vi "ZenCAM Output.vi"(8 "error in (no error)":errorcluster, 9 "Output Data":T1, 10 "State":string, 11 "Camera Controller in":refnum<class "Camera Controller.lvclass">) -> (0 "error out":errorcluster, 3 "Camera Controller out":refnum<class "Camera Controller.lvclass">)   [LabVIEW 2019, in "Camera Controller.lvlib" / "Camera Controller.lvclass"]
uses:
  Camera Controller.lvclass
  <vilib>/ActorFramework/Actor/Actor.lvclass
  <vilib>/vision/Image Controls.llb/IMAQ Image.ctl
  Rack Controller/Rack Controller Messages/CameraOpticsDiagnosticsResult_RC Msg/Camera Optics Diagnostics Result_RC Msg.lvclass
  Rack Controller/Rack Controller Messages/Acknowledgement_RC Msg/Acknowledgement_RC Msg.lvclass
  Rack Controller/Rack Controller Messages/Clear_RC Msg/Clear_RC Msg.lvclass
  Algorithm/Algorithm Messages/ImagesAndCount_Algo Msg/ImagesAndCount_Algo Msg.lvclass
  Rack Controller/Rack Controller Messages/Global Count Value Change_RC Msg/Current Trigger Count_RC Msg.lvclass
  Rack Controller/Rack Controller Messages/Camera Info_RC Msg/Camera Info_RC Msg.lvclass
  Rack Controller/Rack Controller Messages/SensorDiagnosticsResult_RC Msg/SensorDiagnosticsResult_RC Msg.lvclass
  Rack Controller/Rack Controller Messages/Error Message_RC Msg/Error Message_RC Msg.lvclass
  C:/Program Files/National Instruments/LabVIEW 2019/vi.lib/ActorFramework/Actor/Actor.lvclass
  <vilib>/ActorFramework/Message Enqueuer/Message Enqueuer.lvclass
  TypeDef/Output Data.ctl
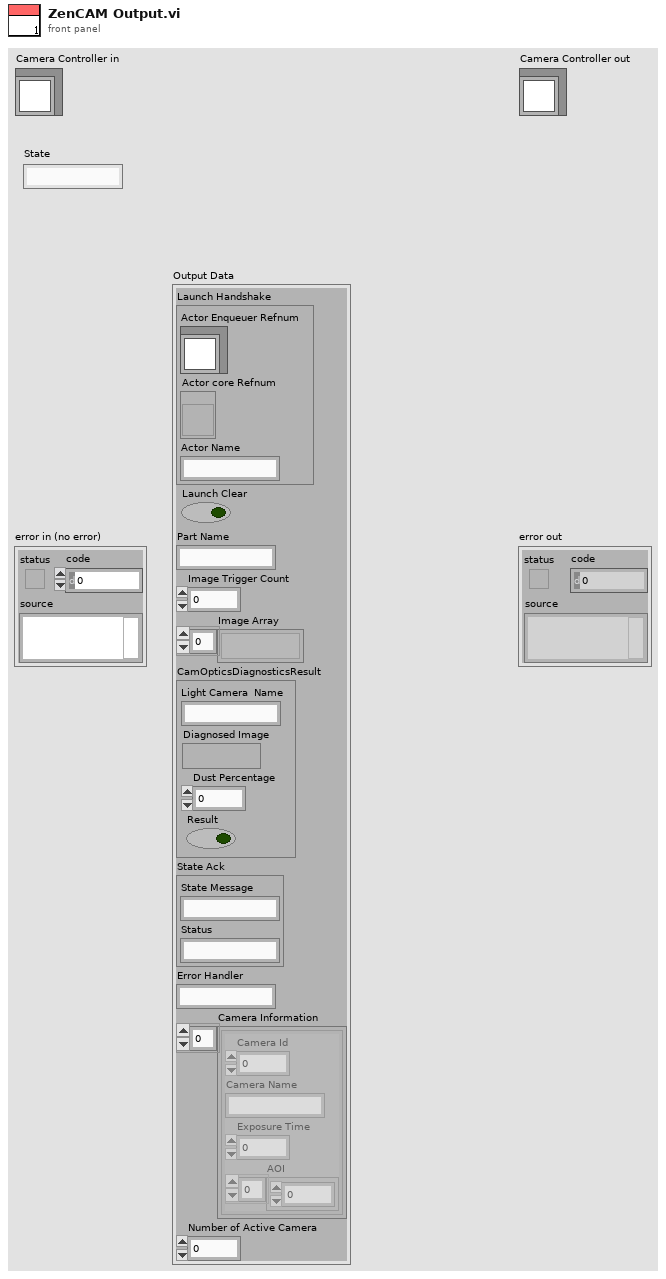
[diagram p1: front panel]
types:
  T1 = typedef "Camera Controller.lvlib/Camera Controller.lvclass/Output Data.ctl" = cluster{"Launch Handshake":cluster{"Actor Enqueuer Refnum":refnum<class "Message Enqueuer.lvclass">, "Actor core Refnum":refnum<vi>, "Actor Name":string}, "Launch Clear":bool, "Part Name":string, "Image Trigger Count":u64, "Image Array":T2[], "CamOpticsDiagnosticsResult":cluster{"Light Camera  Name":string, "Diagnosed Image":T2, "Dust Percentage":dbl, "Result":bool}, "State Ack":cluster{"State Message":string, "Status":string}, "Error Handler":string, "Camera Information":cluster{"Camera Id":i32, "Camera Name":string, "Exposure Time":i32, "AOI":i32[]}[], "Number of Active Camera":i32}
  T2 = typedef "IMAQ Image.ctl" = refnum<image>
  T3 = cluster{"Camera Names":string[], "No. of Active Cameras":u8}
  T4 = cluster{"Actor Enqueuer Refnum":refnum<class "Message Enqueuer.lvclass">, "Actor core Refnum":refnum<vi>, "Actor Name":string}
  T5 = cluster{"Camera Id":i32, "Camera Name":string, "Exposure Time":i32, "AOI":i32[]}[]
  T6 = cluster{"Light Camera  Name":string, "Diagnosed Image":T2, "Dust Percentage":dbl, "Result":bool}
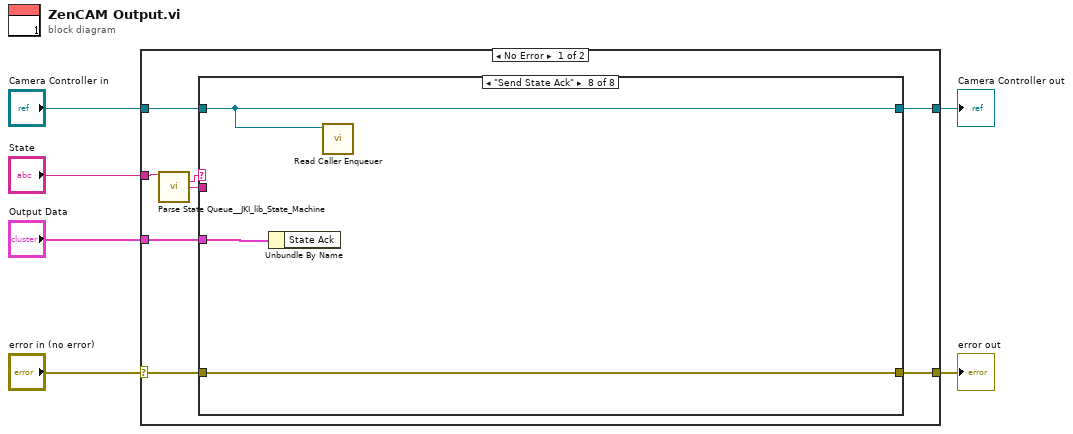
[diagram p0: block diagram]
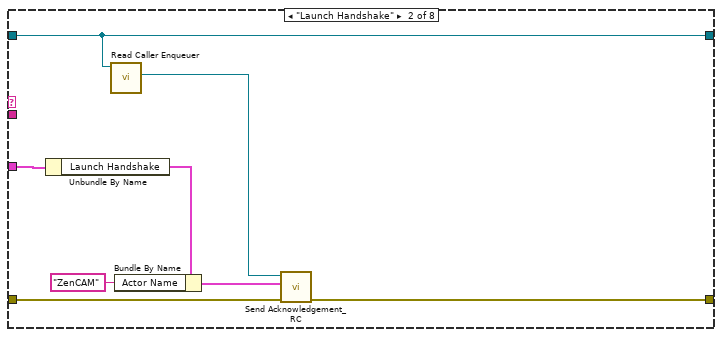
[diagram p3: hidden frame]
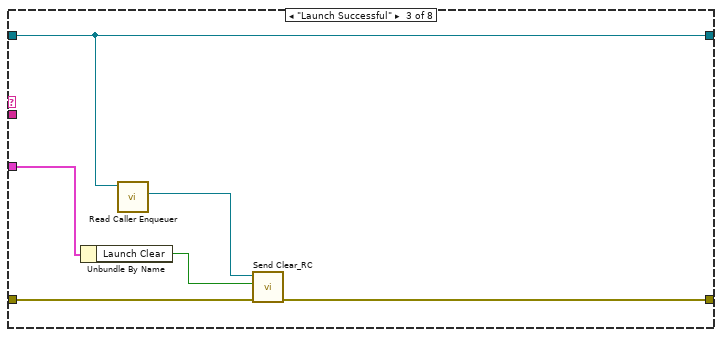
[diagram p4: hidden frame]
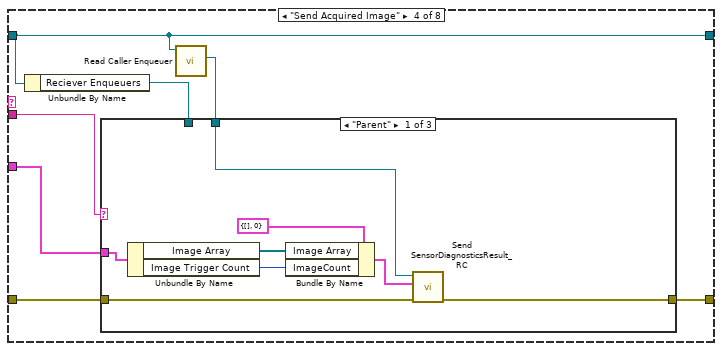
[diagram p5: hidden frame]
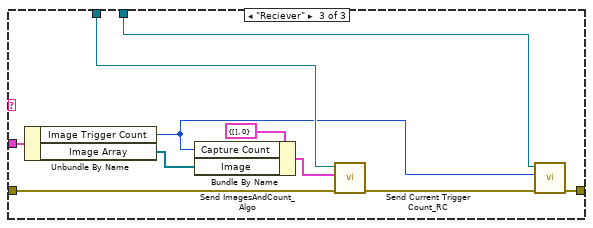
[diagram p7: hidden frame]
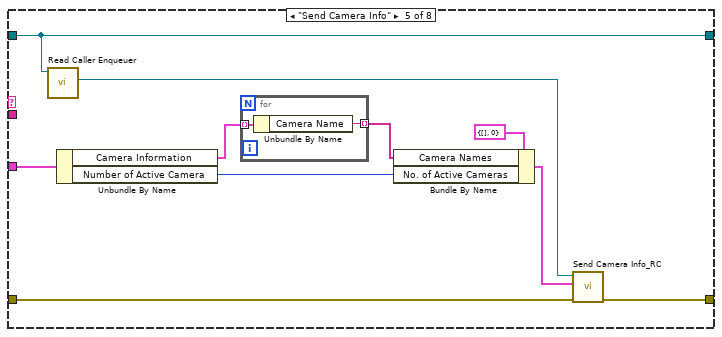
[diagram p8: hidden frame]
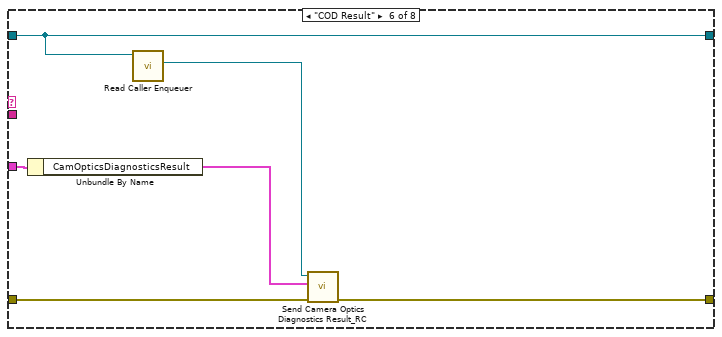
[diagram p9: hidden frame]
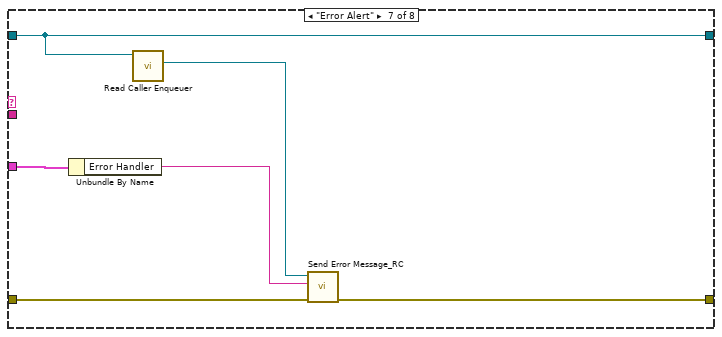
[diagram p10: hidden frame]
diagram:
  n1 = case shown="No Error" "error in (no error)" {
    selector: "error in (no error)" -> [w11 w85]
    tunnel: [w10 w85] -> w5
    tunnel: [w12 w84] -> w3
    tunnel: "Camera Controller in" -> [w13 w84]
    tunnel: "State" -> [w9 _]
    tunnel: "Output Data" -> [w14 _]
    frame No Error {
      n2 = call <vilib>:"Parse State Queue__JKI_lib_State_Machine.vi"("State Queue"=w9) -> ("Current State"=w8:string, "Arguments"=w7:string)  [unwired: 12 in, 1 out]
      n3 = case shown="\"Send State Ack\"" w8 {
        tunnel: w14 -> [_ w24 w30 w37 w66 w74 w80 w83]
        tunnel: w11 -> [w15 w21 w26 w35 w58 w72 w76 w81]
        tunnel: w13 -> [w16 w23 w29 w32 w61 w73 w79 w82]
        tunnel: [w16 w23 w29 w32 w61 w73 w79 w82] -> w12
        tunnel: [w15 w20 w25 w34 w57 w69 w75 w81] -> w10
        tunnel: w7 -> [_ _ _ w33 _ _ _ _]
        frame Default {
        }
        frame "Launch Handshake" {
          n4 = Unbundle By Name(w24) -> ("Launch Handshake"=w19:T4)
          n5 = call <vilib>:"Read Caller Enqueuer.vi"("Actor"=w23) -> ("Caller Enqueuer"=w22:refnum<class "Message Enqueuer.lvclass">)  [unwired: 10 in]
          n6 = Bundle By Name(cluster=w19, "Actor Name"="ZenCAM") -> (w18:T4)
          n7 = call "Send Acknowledgement_RC.vi"("error in (no error)"=w21, "Acknowledgement_RC"=w18, "Message Enqueuer"=w22) -> ("error out"=w20:errorcluster)  [unwired: 7 in, 1 out]
        }
        frame "Launch Successful" {
          n8 = Unbundle By Name(w30) -> ("Launch Clear"=w28:bool)
          n9 = call <vilib>:"Read Caller Enqueuer.vi"("Actor"=w29) -> ("Caller Enqueuer"=w27:refnum<class "Message Enqueuer.lvclass">)  [unwired: 10 in]
          n10 = call "Send Clear_RC.vi"("error in (no error)"=w26, "Clear_RC"=w28, "Message Enqueuer"=w27) -> ("error out"=w25:errorcluster)  [unwired: 7 in, 1 out]
        }
        frame "Send Acquired Image" {
          n11 = Unbundle By Name(w32) -> ("Reciever Enqueuers"=w36:refnum<class "Message Enqueuer.lvclass">)
          n12 = call <vilib>:"Read Caller Enqueuer.vi"("Actor"=w32) -> ("Caller Enqueuer"=w31:refnum<class "Message Enqueuer.lvclass">)  [unwired: 10 in]
          n13 = case shown="\"Parent\"" w33 {
            tunnel: w37 -> [w40 _ w56]
            tunnel: w36 -> [_ _ w52]
            tunnel: w35 -> [w45 w46 w51]
            tunnel: [w44 w46 w49] -> w34
            tunnel: w31 -> [w43 _ w48]
            frame "Parent" {
              n14 = Unbundle By Name(w40) -> ("Image Array"=w39:T2[], "Image Trigger Count"=w38:u64)
              n15 = Bundle By Name(cluster=cluster{"Image Array":T2[], "ImageCount":u64} {"Image Array"=[], "ImageCount"=0} ("ImagesAndCount"), "Image Array"=w39, "ImageCount"=w38) -> (w41:cluster{"Image Array":T2[], "ImageCount":u64})
              n16 = call "Send SensorDiagnosticsResult_RC.vi"("error in (no error)"=w45, "ImagesAndCount"=w41, "Message Enqueuer"=w43) -> ("error out"=w44:errorcluster)  [unwired: 7 in, 1 out]
            }
            frame Default {
            }
            frame "Reciever" {
              n17 = Unbundle By Name(w56) -> ("Image Trigger Count"=w47:u64, "Image Array"=w54:T2[])
              n18 = Bundle By Name(cluster=cluster{"Image":T2[], "Capture Count":u64} {"Image"=[], "Capture Count"=0} ("Captured Image"), "Capture Count"=w47, "Image"=w54) -> (w53:cluster{"Image":T2[], "Capture Count":u64})
              n19 = call "Send ImagesAndCount_Algo.vi"("error in (no error)"=w51, "ImagesAndCount"=w53, "Message Enqueuer"=w52) -> ("error out"=w50:errorcluster)  [unwired: 7 in, 1 out]
              n20 = call "Send Current Trigger Count_RC.vi"("error in (no error)"=w50, "Numeric"=w47, "Message Enqueuer"=w48) -> ("error out"=w49:errorcluster)  [unwired: 7 in, 1 out]
            }
          }
        }
        frame "Send Camera Info" {
          n21 = call <vilib>:"Read Caller Enqueuer.vi"("Actor"=w61) -> ("Caller Enqueuer"=w59:refnum<class "Message Enqueuer.lvclass">)  [unwired: 10 in]
          n22 = Unbundle By Name(w66) -> ("Camera Information"=w65:T5, "Number of Active Camera"=w62:i32)
          n23 = for {
            tunnel: w65 -> [w68] mode=indexing
            tunnel: [w67] -> w63 mode=indexing
            n24 = Unbundle By Name(w68) -> ("Camera Name"=w67:string)
          }
          n25 = Bundle By Name(cluster=T3 {"Camera Names"=[], "No. of Active Cameras"=0} ("Camera Info"), "Camera Names"=w63, "No. of Active Cameras"=w62) -> (w60:T3)
          n26 = call "Send Camera Info_RC.vi"("error in (no error)"=w58, "Camera Info"=w60, "Message Enqueuer"=w59) -> ("error out"=w57:errorcluster)  [unwired: 7 in, 1 out]
        }
        frame "COD Result" {
          n27 = Unbundle By Name(w74) -> ("CamOpticsDiagnosticsResult"=w71:T6)
          n28 = call <vilib>:"Read Caller Enqueuer.vi"("Actor"=w73) -> ("Caller Enqueuer"=w70:refnum<class "Message Enqueuer.lvclass">)  [unwired: 10 in]
          n29 = call "Send Camera Optics Diagnostics Result_RC.vi"("error in (no error)"=w72, "Camera Optics Diagnostics Result"=w71, "Message Enqueuer"=w70) -> ("error out"=w69:errorcluster)  [unwired: 7 in, 1 out]
        }
        frame "Error Alert" {
          n30 = Unbundle By Name(w80) -> ("Error Handler"=w78:string)
          n31 = call <vilib>:"Read Caller Enqueuer.vi"("Actor"=w79) -> ("Caller Enqueuer"=w77:refnum<class "Message Enqueuer.lvclass">)  [unwired: 10 in]
          n32 = call "Send Error Message_RC.vi"("error in (no error)"=w76, "Error Message_RC"=w78, "Message Enqueuer"=w77) -> ("error out"=w75:errorcluster)  [unwired: 7 in, 1 out]
        }
        frame "Send State Ack" {
          n33 = Unbundle By Name(w83) -> ()  [unwired: 1 out]
          n34 = call <vilib>:"Read Caller Enqueuer.vi"("Actor"=w82) -> ()  [unwired: 10 in, 1 out]
        }
      }
    }
    frame Error {
    }
  }
  "error out" <- w5
  "Camera Controller out" <- w3
